vi "macro_vecBuilder7x1FIll.vi"   [LabVIEW 2019, in "Trajectory_Library.lvlib"]
uses:
  MatBuilder_Create.vi
  Trajectory_Library.lvlib
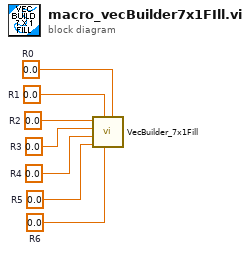
[diagram p0: block diagram]
diagram:
  w1 = 0.0  # R6
  w2 = 0.0  # R5
  w3 = 0.0  # R4
  w4 = 0.0  # R3
  w5 = 0.0  # R2
  w6 = 0.0  # R1
  w7 = 0.0  # R0
  n1 = call "VecBuilder_7x1Fill.vi"("R0"=w7, "R6"=w1, "R1"=w6, "R5"=w2, "R4"=w3, "R3"=w4, "R2"=w5) -> ()  [unwired: 4 in, 1 out]
